vi "SEA_CURRENT_CONTROL_PI_REFERENCE_TEST.vi"() -> ()   [LabVIEW 2019]
uses:
  <vilib>/Platform/TimedLoop/XDataNode/timing_clust.ctl
  <vilib>/Platform/TimedLoop/XDataNode/nitl_modes.ctl
  <vilib>/Platform/TimedLoop/XDataNode/wakeup.ctl
  <vilib>/FPGAPlugInAG/sbRIO-9627/niLvFpga_Open_sbRIO-9627.vi
  <vilib>/rvi/interface/common/dynamic/niFpgaDynamicAddResources.vi
  <vilib>/Utility/error.llb/Error Cluster From Error Code.vi
  <vilib>/rvi/errors/niLvFpgaAdjustHostInterfaceError.vi
  <vilib>/RVI Host/nirviSupport.llb/nirviErrorClusterFromErrorCode.vi
  <vilib>/FPGAPlugInAG/Dynamic/niLvFpga_Close_Dynamic.vi
  <vilib>/rvi/interface/nirviOpenFPGA/nirviOpenFPGA.xnode
  FPGA Bitfiles/seafinalexperime_FPGATarget_SEACURRENTCONTRO_63doizOrvmw.lvbitx
  SEA_CURRENT_CONTROL_PI.vi
  <vilib>/platform/TimedLoop/XDataNode/XDataNode.xnode
  <vilib>/rvi/interface/nirviMethod/nirviMethod.xnode
  <vilib>/rvi/interface/nirviReadWriteControl/nirviReadWriteControl.xnode
  <vilib>/rvi/interface/nirviCloseFPGA/nirviCloseFPGA.xnode
  NiFpgaLv.dll
  <vilib>/rvi/interface/Simulation/niFpgaSimulationCallBeginRW.vi
  <vilib>/Platform/TimedLoop/XDataNode/XDNodeRunTimeDep.lvlib
  <vilib>/FPGAPlugInAG/Dynamic/niLvFpga_ReadFifo_Dynamic.vi
  <vilib>/rvi/errors/niLvFpgaMergeErrorWithErrorCode.vi
  <vilib>/FPGAPlugInAG/Dynamic/niLvFpga_WriteFifo_Dynamic.vi
  <vilib>/rvi/interface/nirviMethod/StockFPGA_InlinedMethodWaitForSingleIRQ.vi
  <vilib>/FPGAPlugInAG/Dynamic/niLvFpga_WaitOnIrq_Dynamic.vi
  <vilib>/FPGAPlugInAG/Dynamic/niLvFpga_AcknowledgeIrq_Dynamic.vi
panel:
  out "Waveform Chart":dynamicdata(graph)
  in  "Ki":sgl
  out "Motor Direction":bool
  in  "Kp":sgl
  out "Current error %":sgl(knob) scale=-100.0..100.0
  in  "Current Offset":sgl
  out "Finished late":u32
  out "Overflow count":u32
  out "Flushed data":sgl[](array[numeric])
  in  "Amplitude":sgl
  in  "frequency":sgl
  in  "stop":bool
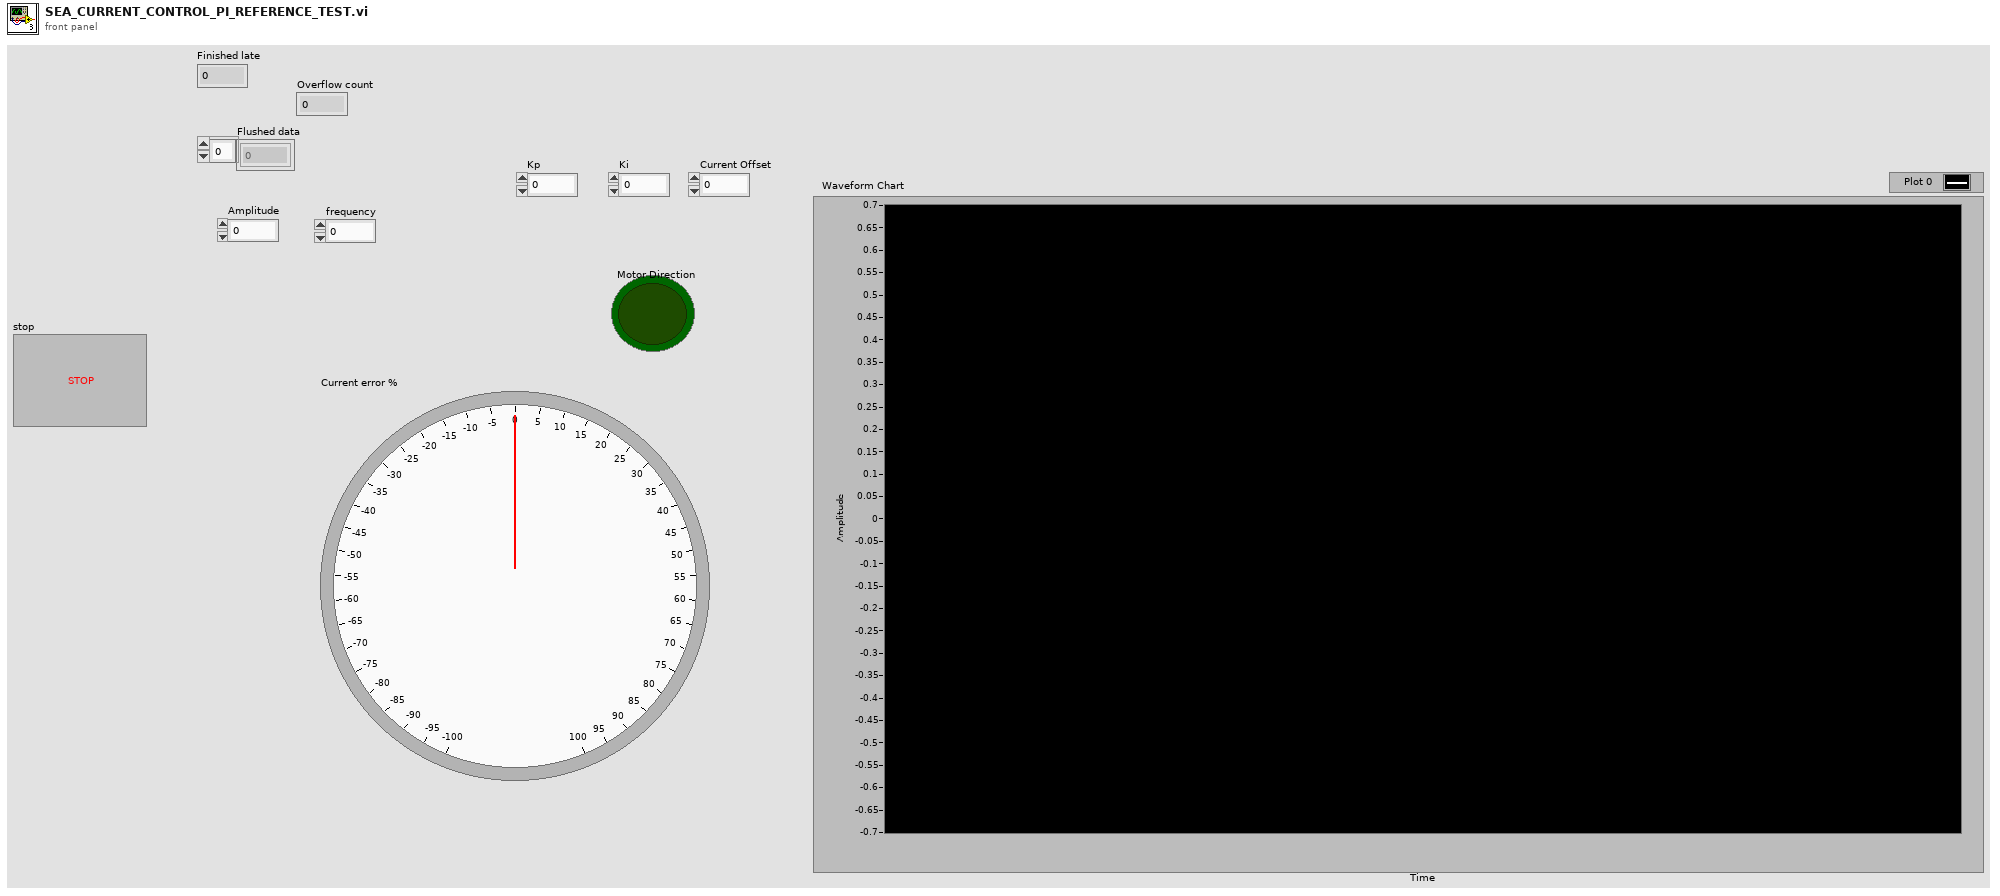
[diagram p1: front panel]
types:
  T1 = typedef "XDNodeRunTimeDep.lvlib/timing_clust.ctl" = cluster{"Expected End [f-1]":u64, "Actual End [f-1]":u64, "Finished Late? [f-1]":bool, "Expected End [i-1]":u64, "Actual End [i-1]":u64, "Finished Late? [i-1]":bool, "Expected Start [i]":u64, "Actual Start [i]":u64, "Expected Start [f]":u64, "Actual Start [f]":u64, "Source Name":string, "Structure Name":string, "Period":i64, "Deadline":i64, "Offset":i64, "Start":i64, "Priority":i32, "Timeout":i32, "Mode":T2, "Wakeup Reason":T3, "Error":errorcluster, "Source Type":string, "Secondary Source Type":string, "Global End Time":u64, "Global Start Time":u64, "Frame Duration":u64, "Iteration Duration":u64, "Assigned CPU":i32, "I/O Scan Engine Mode":u32}
  T2 = typedef "XDNodeRunTimeDep.lvlib/nitl_modes.ctl" = enum32{"No Change", "Process missed periods, maintain original phase", "Discard missed periods, maintain original phase", "Process missed periods, ignore original phase", "Discard missed periods, ignore original phase"}
  T3 = typedef "XDNodeRunTimeDep.lvlib/wakeup.ctl" = enum32{"Normal", "Aborted", "Asynchronous wakeup", "Timing source error", "Timed loop error", "Timeout"}
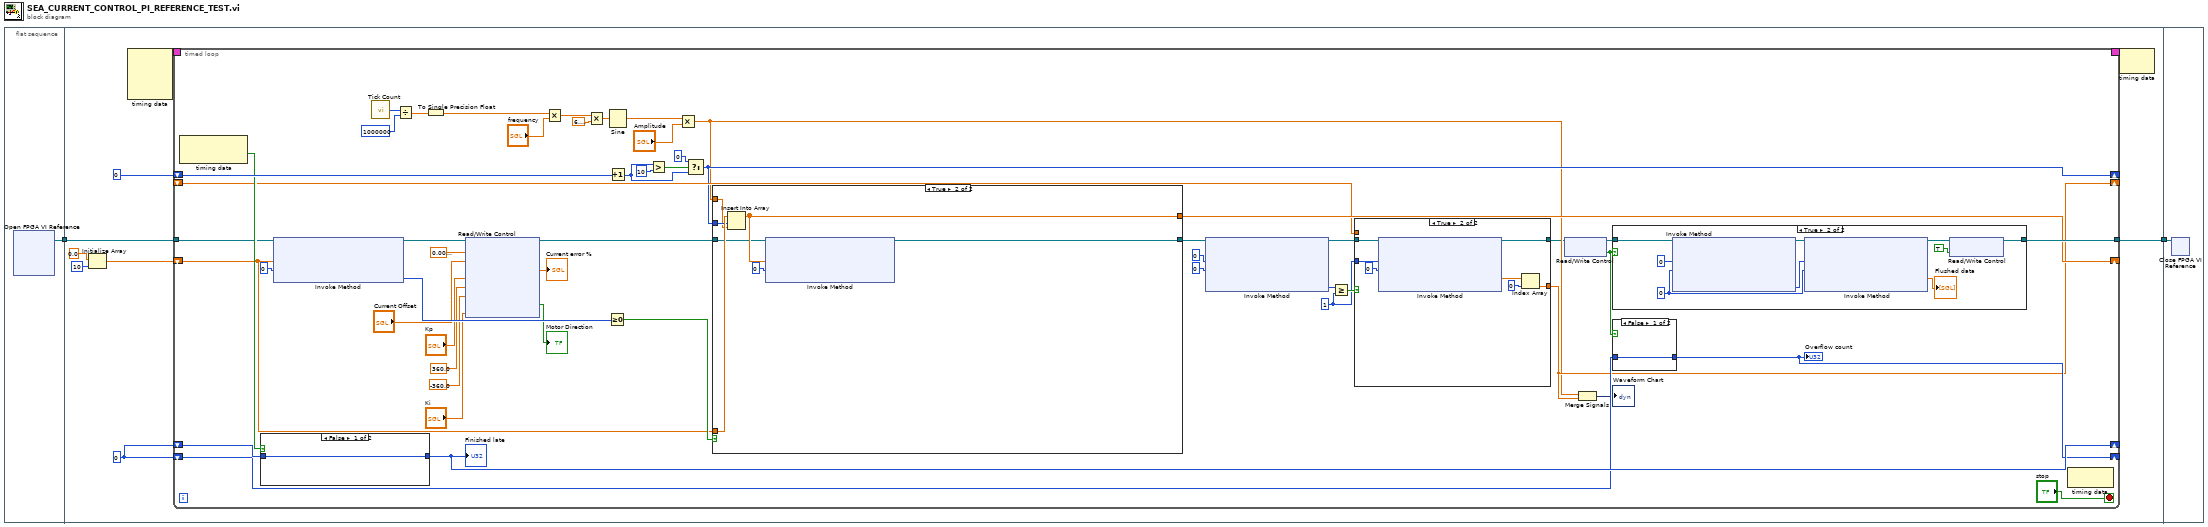
[diagram p0: block diagram]
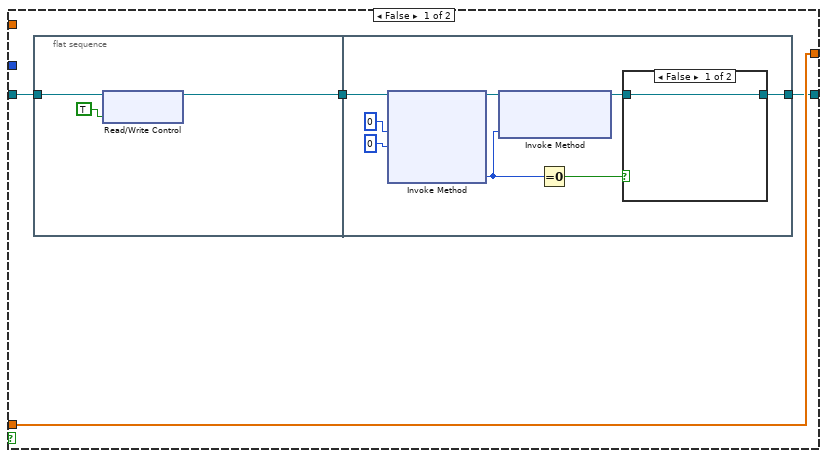
[diagram p2: hidden frame]
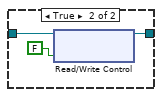
[diagram p3: hidden frame]
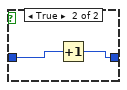
[diagram p4: hidden frame]
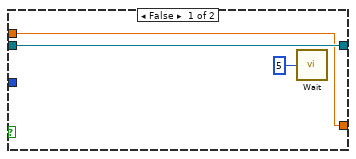
[diagram p6: hidden frame]
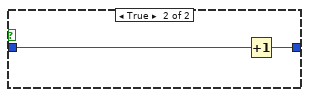
[diagram p7: hidden frame]
diagram:
  n1 = flat-sequence {
    tunnel: [w3] -> w2
    tunnel: w2 -> [w12]
    tunnel: [w9] -> w1
    tunnel: w1 -> [w123]
    frame #0 {
      n2 = xnode "Open FPGA VI Reference"() -> ("FPGA VI Reference Out"=w3:refnum<k20>)  [unwired: 2 in, 1 out]
    }
    frame #1 {
      w8 = u32 0
      n3 = Initialize Array(sgl 0.0 ("element"), 10 ("dimension size")) -> (w4:sgl[])
      n4 = node-c288() -> (w11:T1)  [unwired: 4 in]
      n5 = timed-loop {
        tunnel: w12 -> [w31]
        timing: w11 -> [_]
        timing-out: [_] -> w10
        shift-right: [w53] -> _
        shift-left: w8 -> [w54]
        tunnel: [w46] -> w9
        shift-right: [w43] -> _
        shift-left: w8 -> [w44]
        shift-right: [w27] -> _
        shift-left: i8 0 -> [w41]
        shift-right: [w32] -> _
        shift-left: w4 -> [w33]
        shift-right: [w17] -> _
        shift-left: _ -> [w28]
        stop <- "stop" stop-if-true
        w47 = u32 1 ("y")
        n6 = node-c288() -> (w35:bool)  [unwired: 1 in, 1 out]
        n7 = case shown="False" w35 {
          tunnel: w54 -> [w115 w117]
          tunnel: [w115 w116] -> w53
          frame False {
          }
          frame True {
            n8 = Increment(x=w117) -> (x+1=w116:u32)
          }
        }
        "Finished late" <- w53
        n9 = xnode "Invoke Method"("FPGA VI Reference In"=w31, "Data"=w33, "Timeout (ms)"=0) -> ("FPGA VI Reference Out"=w14:refnum<k20>, "Empty Elements Remaining"=w36:u32)  [unwired: 1 in, 1 out]
        n10 = call "Tick Count"() -> ("Tick Count(uSec)"=w64:u32)
        n11 = Divide(x=w64, y=u32 1000000) -> (x/y=w61:dbl)
        n12 = To Single Precision Float(number=w61) -> (single precision float=w62:sgl)
        n13 = xnode "Read/Write Control"("FPGA VI Reference In"=w14, "weighting term(M2)"=sgl 0.01, "Current Offset"="Current Offset", "Kp"="Kp", "UB"=sgl 360.0, "LB"=sgl -360.0, "Ki"="Ki") -> ("FPGA VI Reference Out"=w15:refnum<k20>, "Current error %"=→"Current error %":sgl, "Motor Direction"=→"Motor Direction":bool)  [unwired: 1 in, 1 out]
        n14 = Multiply(x=w62, y="frequency") -> (x*y=w60:sgl)
        n15 = Multiply(x=w60, y=sgl 6.2831855) -> (x*y=w58:sgl)
        n16 = Greater Or Equal To 0?(x=w36) -> (x >= 0?=w34:bool)
        n17 = Sine(x=w58) -> (sin(x)=w56:sgl)
        n18 = Increment(x=w41) -> (x+1=w37:i8)
        n19 = Greater?(x=w37, y=i8 10) -> (0:w39:bool)
        n20 = Multiply(x=w56, y="Amplitude") -> (x*y=w16:sgl)
        n21 = Select(t=i8 0, s=w39, f=w37) -> (s? t:f=w27:i8)
        n22 = case shown="True" w34 {
          tunnel: w33 -> [w69 w91]
          tunnel: w27 -> [_ w90]
          tunnel: w16 -> [_ w89]
          tunnel: [w69 w88] -> w32
          tunnel: w15 -> [w68 w86]
          tunnel: [w66 w85] -> w30
          frame False {
            n23 = flat-sequence {
              tunnel: w68 -> [w72]
              tunnel: [w70] -> w67
              tunnel: w67 -> [w77]
              tunnel: [w73] -> w66
              frame #0 {
                n24 = xnode "Read/Write Control"("FPGA VI Reference In"=w72, "RT overflow"=TRUE) -> ("FPGA VI Reference Out"=w70:refnum<k20>)  [unwired: 1 in, 1 out]
              }
              frame #1 {
                n25 = xnode "Invoke Method"("FPGA VI Reference In"=w77, "IRQ Number(s)"=0, "Timeout (ms)"=0) -> ("FPGA VI Reference Out"=w78:refnum<k20>, "IRQ(s) Asserted"=w76:i32)  [unwired: 1 in, 2 out]
                n26 = xnode "Invoke Method"("FPGA VI Reference In"=w78, "IRQ Number(s)"=w76) -> ("FPGA VI Reference Out"=w74:refnum<k20>)  [unwired: 1 in, 1 out]
                n27 = Equal To 0?(x=w76) -> (x = 0?=w75:bool)
                n28 = case shown="False" w75 {
                  tunnel: w74 -> [w81 w84]
                  tunnel: [w81 w83] -> w73
                  frame False {
                  }
                  frame True {
                    n29 = xnode "Read/Write Control"("FPGA VI Reference In"=w84, "RT overflow"=FALSE) -> ("FPGA VI Reference Out"=w83:refnum<k20>)  [unwired: 1 in, 1 out]
                  }
                }
              }
            }
          }
          frame True {
            n30 = Insert Into Array(array=w91, index=w90, new element=w89) -> (w88:sgl[])
            n31 = xnode "Invoke Method"("FPGA VI Reference In"=w86, "Data"=w88, "Timeout (ms)"=0) -> ("FPGA VI Reference Out"=w85:refnum<k20>)  [unwired: 1 in, 2 out]
          }
        }
        n32 = xnode "Invoke Method"("FPGA VI Reference In"=w30, "Number of Elements"=u32 0, "Timeout (ms)"=0) -> ("FPGA VI Reference Out"=w48:refnum<k20>, "Elements Remaining"=w50:u32)  [unwired: 1 in, 2 out]
        n33 = Greater Or Equal?(x=w50, y=w47) -> (x >= y?=w49:bool)
        n34 = case shown="True" w49 {
          tunnel: w48 -> [w106 w114]
          tunnel: w47 -> [_ w113]
          tunnel: [w106 w111] -> w13
          tunnel: [w105 w108] -> w17
          tunnel: w28 -> [w105 _]
          frame False {
            n35 = call "Wait"("Count(uSec)"=u32 5) -> ()  [unwired: 1 out]
          }
          frame True {
            n36 = xnode "Invoke Method"("FPGA VI Reference In"=w114, "Number of Elements"=w113, "Timeout (ms)"=0) -> ("FPGA VI Reference Out"=w111:refnum<k20>, "Data"=w110:sgl[])  [unwired: 1 in, 2 out]
            n37 = Index Array(array=w110, index=0) -> (element=w108:sgl)
          }
        }
        n38 = xnode "Read/Write Control"("FPGA VI Reference In"=w13) -> ("FPGA VI Reference Out"=w29:refnum<k20>, "Overflow?"=w45:bool)  [unwired: 1 in, 1 out]
        n39 = Merge Signals(w16, w17) -> (→"Waveform Chart":dynamicdata)
        n40 = case shown="True" w45 {
          tunnel: w29 -> [w95 w100]
          tunnel: [w95 w96] -> w46
          frame False {
          }
          frame True {
            w101 = 0 ("Timeout (ms)")
            n41 = xnode "Invoke Method"("FPGA VI Reference In"=w100, "Number of Elements"=u32 0, "Timeout (ms)"=w101) -> ("FPGA VI Reference Out"=w99:refnum<k20>, "Elements Remaining"=w103:u32)  [unwired: 1 in, 2 out]
            n42 = xnode "Invoke Method"("FPGA VI Reference In"=w99, "Number of Elements"=w103, "Timeout (ms)"=w101) -> ("FPGA VI Reference Out"=w98:refnum<k20>, "Data"=→"Flushed data":sgl[])  [unwired: 1 in, 2 out]
            n43 = xnode "Read/Write Control"("FPGA VI Reference In"=w98, "DMA cleared?"=TRUE) -> ("FPGA VI Reference Out"=w96:refnum<k20>)  [unwired: 1 in, 1 out]
          }
        }
        n44 = case shown="False" w45 {
          tunnel: w44 -> [w92 w94]
          tunnel: [w92 w93] -> w43
          frame False {
          }
          frame True {
            n45 = Increment(x=w94) -> (x+1=w93:u32)
          }
        }
        "Overflow count" <- w43
        n46 = node-c288() -> ()  [unwired: 1 in, 1 out]
      }
      n47 = node-c288(w10) -> ()  [unwired: 1 out]
    }
    frame #2 {
      n48 = xnode "Close FPGA VI Reference"("FPGA VI Reference In"=w123) -> ()  [unwired: 1 in, 1 out]
    }
  }
